vi "Scan Engine Slot Page.vi"(8 "error in (no error)":errorcluster, 11 "Node Ptr":T1 format="%.0x") -> (0 "error out":errorcluster)   [LabVIEW 2017, in "Scan Engine Custom Device.lvlib"]
uses:
  Scan Engine Custom Device.lvlib
  <vilib>/NI Veristand/Custom Device API/Custom Device Item Ref.ctl
  Modules.lvlibp/RSI Module/SubPanel Command.ctl
  Globals/Scan Engine GUIDs.vi
  <vilib>/NI Veristand/Custom Device API/Custom Device API.lvlib
  Modules.lvlibp/RSI Module/RSI Module.lvclass
panel:
  out "Slot #":u32
  in  "Modules":string(combo)
  in  "Header":cluster{"Section Name":string}={"Section Name"="Slot Settings"}
  in  "Description":string
  out "Name":string
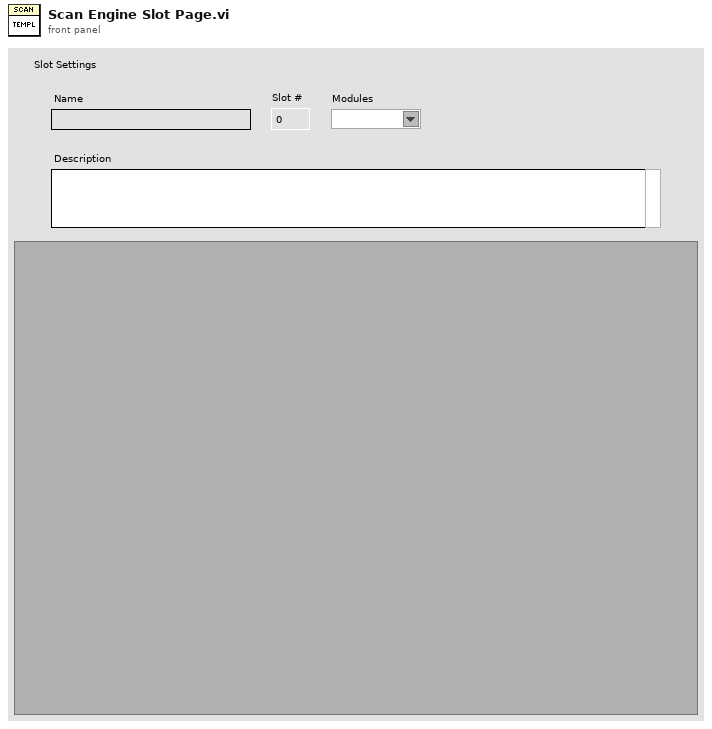
[diagram p1: front panel]
types:
  T1 = typedef "Custom Device API.lvlib/Custom Device Item Ref.ctl" = u64
  T2 = enum8{"Enabled", "Disabled", "Disabled and Grayed Out"}
  T3 = typedef "Custom Device API.lvlib/Custom Device Item Info.ctl" = cluster{"Name":string, "Is Channel":bool, "GUID":string, "Is Waveform":bool}
  T4 = typedef "Modules.lvlibp/RSI Module.lvclass/Module Models.ctl" = enum16{"Empty", "NI 9201", "NI 9203", "NI 9205", "NI 9206", "NI 9207", "NI 9208", "NI 9211", "NI 9212", "NI 9213", "NI 9214", "NI 9215", "NI 9217", "NI 9219", "NI 9220", "NI 9221", "NI 9222", "NI 9223", "NI 9225", "NI 9227", "NI 9229", "NI 9233", "NI 9234", "NI 9235", "NI 9236", "NI 9237", "NI 9239", "NI 9242", "NI 9244", "NI 9263", "NI 9264", "NI 9265", "NI 9269", "NI 9375", "NI 9401", "NI 9402", "NI 9403", "NI 9411", "NI 9421", "NI 9422", "NI 9423", "NI 9425", "NI 9426", "NI 9435", "NI 9437", "NI 9472", "NI 9474", "NI 9475", "NI 9476", "NI 9477", "NI 9478", "NI 9481", "NI 9482", "NI 9485", "NI 9266"}
  T5 = typedef "Modules.lvlibp/RSI Module.lvclass/SubPanel Command.ctl" = enum16{"Stop"}
  T6 = typedef "Custom Device API.lvlib/Custom Device Commands.ctl" = enum16{"Default", "Item renamed", "Shutdown", "Dynamic button pressed"}
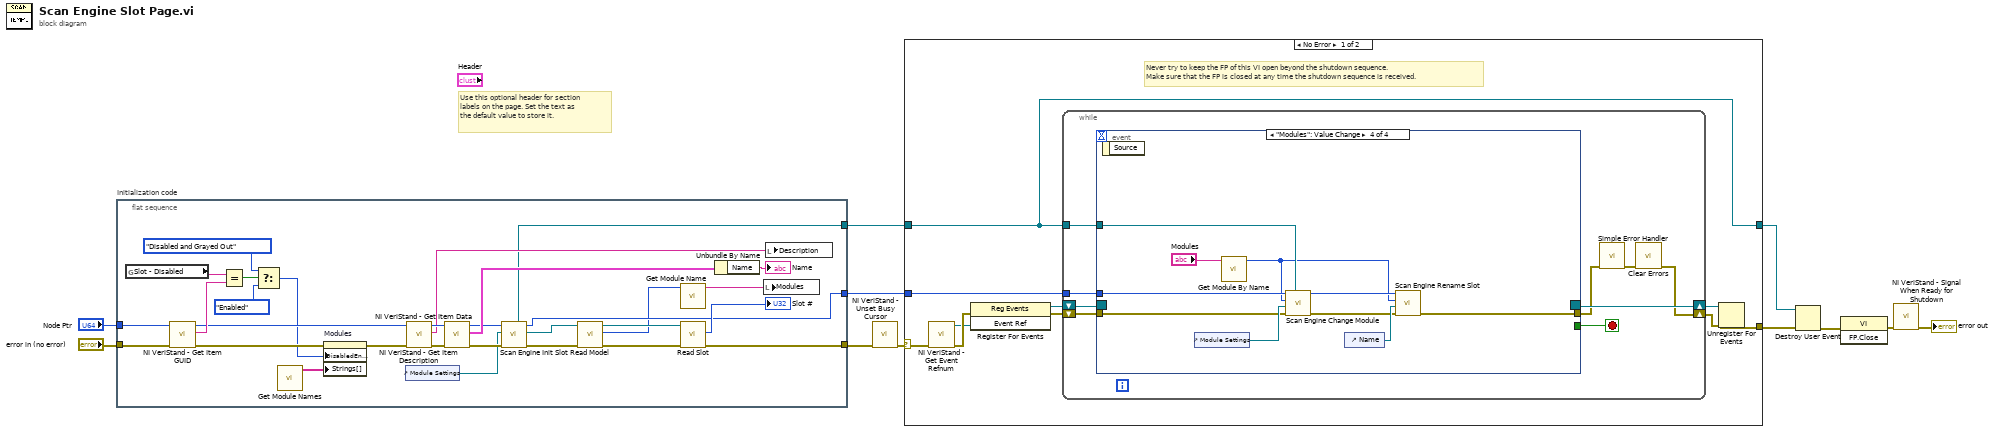
[diagram p0: block diagram]
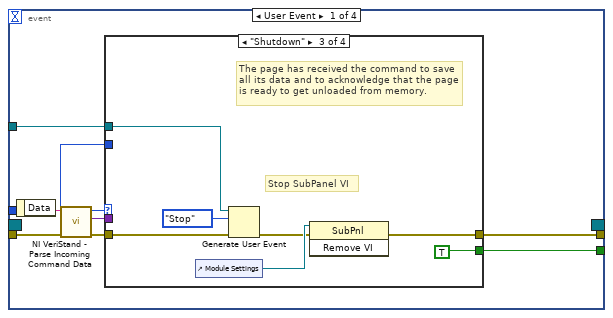
[diagram p2: hidden frame]
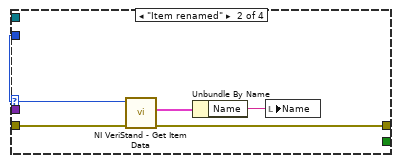
[diagram p4: hidden frame]
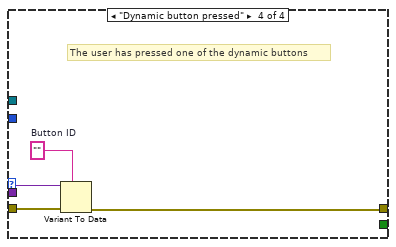
[diagram p5: hidden frame]
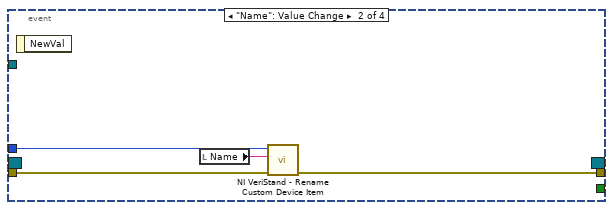
[diagram p6: hidden frame]
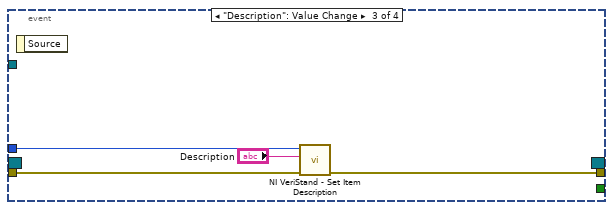
[diagram p7: hidden frame]
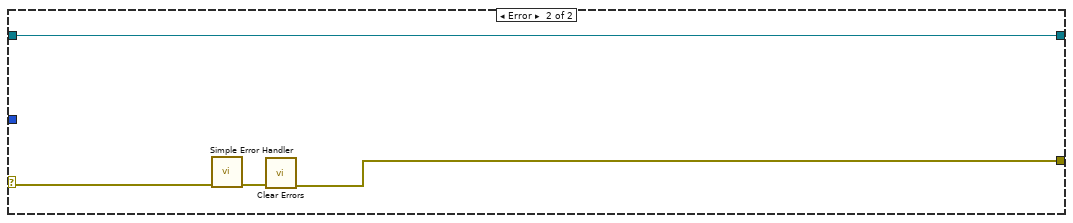
[diagram p8: hidden frame]
diagram:
  # "Use this optional header for section labels on the page. Set the text as the default value to store it."
  n1 = flat-sequence "Initialization code" {
    tunnel: "error in (no error)" -> [w24]
    tunnel: "Node Ptr" -> [w25]
    tunnel: [w26] -> w8
    tunnel: [w28] -> w5
    tunnel: [w30] -> w4
    frame #0 {
      n2 = global read "Scan Engine GUIDs.vi" "Slot - Disabled"() -> (w23:string)
      n3 = call <vilib>:"NI VeriStand - Get Item GUID.vi"("error in (no error)"=w24, "Item Ref in"=w25) -> ("error out"=w15:errorcluster, "GUID"=w22:string, "Item Ref out"=w21:T1)  [unwired: 7 in]
      n4 = Equal?(x=w23, y=w22) -> (x = y?=w20:bool)
      n5 = Select(t=T2."Disabled and Grayed Out" ("Disabled"), s=w20, f=T2."Enabled" ("Disabled")) -> (s? t:f=w13:T2)
      n6 = call "Get Module Names.vi"() -> ("Module Names"=w14:string[])  [unwired: 11 in]
      n7 = property on="Modules" class="CmbBox"(error in=w15, "DisabledEnum"=w13, "Strings[]"=w14) -> (error out=w12:errorcluster)  [unwired: 1 in, 1 out]
      n8 = control-ref of="Module Settings"() -> (w31:refnum<vi>)
      n9 = call <vilib>:"NI VeriStand - Get Item Description.vi"("error in (no error)"=w12, "Item Ref in"=w21) -> ("error out"=w39:errorcluster, "Description"=w40:string, "Item Ref out"=w41:T1)  [unwired: 7 out]
      n10 = call <vilib>:"NI VeriStand - Get Item Data.vi"("error in (no error)"=w39, "Item Ref in"=w41) -> ("error out"=w33:errorcluster, "Item Info"=w38:T3, "Item Ref out"=w32:T1)  [unwired: 7 out]
      n11 = call "Scan Engine Init Slot.vi"("error in (no error)"=w33, "SubPanel Ref"=w31, "Node Ptr In"=w32) -> ("error out"=w27:errorcluster, "RSI Module"=w29:refnum<class "RSI Module.lvclass">, "Node Ptr Out"=w28:T1, "SubPanel Command"=w30:refnum<user-event>)  [unwired: 5 in]
      n12 = call "Read Model.vi"("error in (no error)"=w27, "RSI Module in"=w29) -> ("error out"=w35:errorcluster, "Model"=w17:T4, "RSI Module out"=w36:refnum<class "RSI Module.lvclass">)  [unwired: 7 in]
      n13 = call "Get Module Name.vi"("Module"=w17) -> ("Module Name"=w16:string)  [unwired: 10 in]
      n14 = call "Read Slot.vi"("error in (no error)"=w35, "RSI Module in"=w36) -> ("error out"=w26:errorcluster, "Slot"=→"Slot #":u32)  [unwired: 7 in, 1 out]
      n15 = Unbundle By Name(w38) -> ("Name"=→"Name":string)
      n16 = local write "Modules"(w16) -> ()
      n17 = local write "Description"(w40) -> ()
    }
  }
  n18 = call <vilib>:"NI VeriStand - Unset Busy Cursor.vi"("error in (no error)"=w8) -> ("error out"=w7:errorcluster)  [unwired: 10 out]
  n19 = case shown="No Error" w7 {
    selector: w7 -> [w43 w108]
    tunnel: [w48 w106] -> w2
    tunnel: w5 -> [w44 _]
    tunnel: w4 -> [w42 w105]
    tunnel: [w42 w105] -> w3
    frame No Error {
      # "Never try to keep the FP of this VI open beyond the shutdown sequence.\nMake sure that the FP is closed at any time the shutdown sequence is received."
      n20 = call <vilib>:"NI VeriStand - Get Event Refnum.vi"("error in (no error)"=w43) -> ("error out"=w51:errorcluster, "Event Ref"=w47:refnum<user-event>)  [unwired: 9 out]
      n21 = register-events(error in=w51, w47) -> (reference out=w45:refnum<event-registration>, error out=w46:errorcluster)  [unwired: 1 in]
      n22 = while {
        tunnel: w44 -> [w56]
        shift-right: [w53] -> w49
        shift-left: w46 -> [w59]
        shift-right: [w60] -> w50
        shift-left: w45 -> [w58]
        tunnel: w42 -> [w52]
        stop <- w57 stop-if-true
        n23 = event shown="[3] \"Modules\": Value Change" {
          selector: w58 -> [_ _ _ _]
          dyn-events: [_ _ _ _] -> w60
          timeout: _ -> [_ _ _ _]
          tunnel: w59 -> [w69 w90 w93 w101]
          tunnel: [w65 _ _ _] -> w57
          tunnel: [w64 w89 w92 w97] -> w55
          tunnel: w56 -> [w63 w88 w94 w100]
          tunnel: w52 -> [w61 _ _ w102]
          event User Event {
            n24 = event-data() -> ("Data"=w68:string)  [unwired: 1 out]
            n25 = call <vilib>:"NI VeriStand - Parse Incoming Command Data.vi"("error in (no error)"=w69, "Incoming data"=w68) -> ("error out"=w67:errorcluster, "Outgoing data"=w62:variant, "Action"=w66:T6)  [unwired: 7 out]
            n26 = case shown="\"Shutdown\"" w66 {
              tunnel: w67 -> [w70 w75 w79 w86]
              tunnel: [_ _ TRUE _] -> w65
              tunnel: [w70 w72 w76 w83] -> w64
              tunnel: w63 -> [_ w74 _ _]
              tunnel: w62 -> [_ _ _ w85]
              tunnel: w61 -> [_ _ w81 _]
              frame "Default", Default {
              }
              frame "Item renamed" {
                n27 = call <vilib>:"NI VeriStand - Get Item Data.vi"("error in (no error)"=w75, "Item Ref in"=w74) -> ("error out"=w72:errorcluster, "Item Info"=w73:T3)  [unwired: 8 out]
                n28 = Unbundle By Name(w73) -> ("Name"=w71:string)
                n29 = local write "Name"(w71) -> ()
              }
              frame "Shutdown" {
                # "Stop SubPanel VI"
                # "The page has received the command to save all its data and to acknowledge that the page is ready to get unloaded from memory."
                n30 = control-ref of="Module Settings"() -> (w78:refnum<vi>)
                n31 = Generate User Event(user event=w81, event data cluster=SubPanel_Command."Stop" ("event data"), error in=w79) -> (error out=w77:errorcluster)  [unwired: 1 in, 1 out]
                n32 = invoke class="SubPnl" method="Remove VI"(reference=w78, error in=w77) -> (error out=w76:errorcluster)  [unwired: 1 in, 2 out]
              }
              frame "Dynamic button pressed" {
                w84 = ""  # Button ID
                # "The user has pressed one of the dynamic buttons"
                n33 = Variant To Data(error in=w86, type=w84, Variant=w85) -> (error out=w83:errorcluster)  [unwired: 1 out]
              }
            }
          }
          event "Name": Value Change {
            n34 = event-data() -> ()  [unwired: 2 out]
            n35 = local read "Name"() -> (w87:string)
            n36 = call <vilib>:"NI VeriStand - Rename Custom Device Item.vi"("error in (no error)"=w90, "New Name"=w87, "Item Ref in"=w88) -> ("error out"=w89:errorcluster)  [unwired: 1 in, 7 out]
          }
          event "Description": Value Change {
            n37 = event-data() -> ()  [unwired: 2 out]
            n38 = call <vilib>:"NI VeriStand - Set Item Description.vi"("error in (no error)"=w93, "Description"="Description", "Item Ref in"=w94) -> ("error out"=w92:errorcluster)  [unwired: 8 out]
          }
          event "Modules": Value Change {
            n39 = event-data() -> ()  [unwired: 2 out]
            n40 = control-ref of="Module Settings"() -> (w103:refnum<vi>)
            n41 = call "Get Module By Name.vi"("Module Name"="Modules") -> ("Module"=w95:T4)  [unwired: 10 in]
            n42 = call "Scan Engine Change Module.vi"("SubPanel Event"=w102, "error in (no error)"=w101, "SubPanel Ref"=w103, "Module Model"=w95, "Node Ptr In"=w100) -> ("error out"=w98:errorcluster, "Node Ptr Out"=w99:T1)  [unwired: 5 in]
            n43 = control-ref of="Name"() -> (w104:refnum<vi>)
            n44 = call "Scan Engine Rename Slot.vi"("error in (no error)"=w98, "Name reference"=w104, "Module Model"=w95, "Node Ptr In"=w99) -> ("error out"=w97:errorcluster)  [unwired: 6 in, 1 out]
          }
        }
        n45 = call <vilib>:"Simple Error Handler.vi"("error in (no error)"=w55) -> ("error out"=w54:errorcluster)  [unwired: 1 in, 7 out]
        n46 = call <vilib>:"Clear Errors.vi"("error in (no error)"=w54) -> ("error out"=w53:errorcluster)  [unwired: 1 in, 5 out]
      }
      n47 = Unregister For Events(event registration refnum=w50, error in=w49) -> (error out=w48:errorcluster)
    }
    frame Error {
      n48 = call <vilib>:"Simple Error Handler.vi"("error in (no error)"=w108) -> ("error out"=w107:errorcluster)  [unwired: 1 in, 7 out]
      n49 = call <vilib>:"Clear Errors.vi"("error in (no error)"=w107) -> ("error out"=w106:errorcluster)  [unwired: 1 in, 5 out]
    }
  }
  n50 = Destroy User Event(user event=w3, error in=w2) -> (error out=w1:errorcluster)
  n51 = invoke class="VI" method="FP.Close"(error in=w1) -> (error out=w11:errorcluster)  [unwired: 2 in, 2 out]
  n52 = call <vilib>:"NI VeriStand - Signal When Ready for Shutdown.vi"("error in (no error)"=w11) -> ("error out"=→"error out":errorcluster)  [unwired: 10 out]
